vi "首页.vi"() -> ()   [LabVIEW 2016]
uses:
  <vilib>/Utility/miscctls.llb/LVPointTypeDef.ctl
  PLC/PLC.lvlib
  API/database/SQLite/SQLite Lib.lvlib
  API/database/Access/Access Lib.lvlib
panel:
  out "显示":T1
  out "动力环境":T3
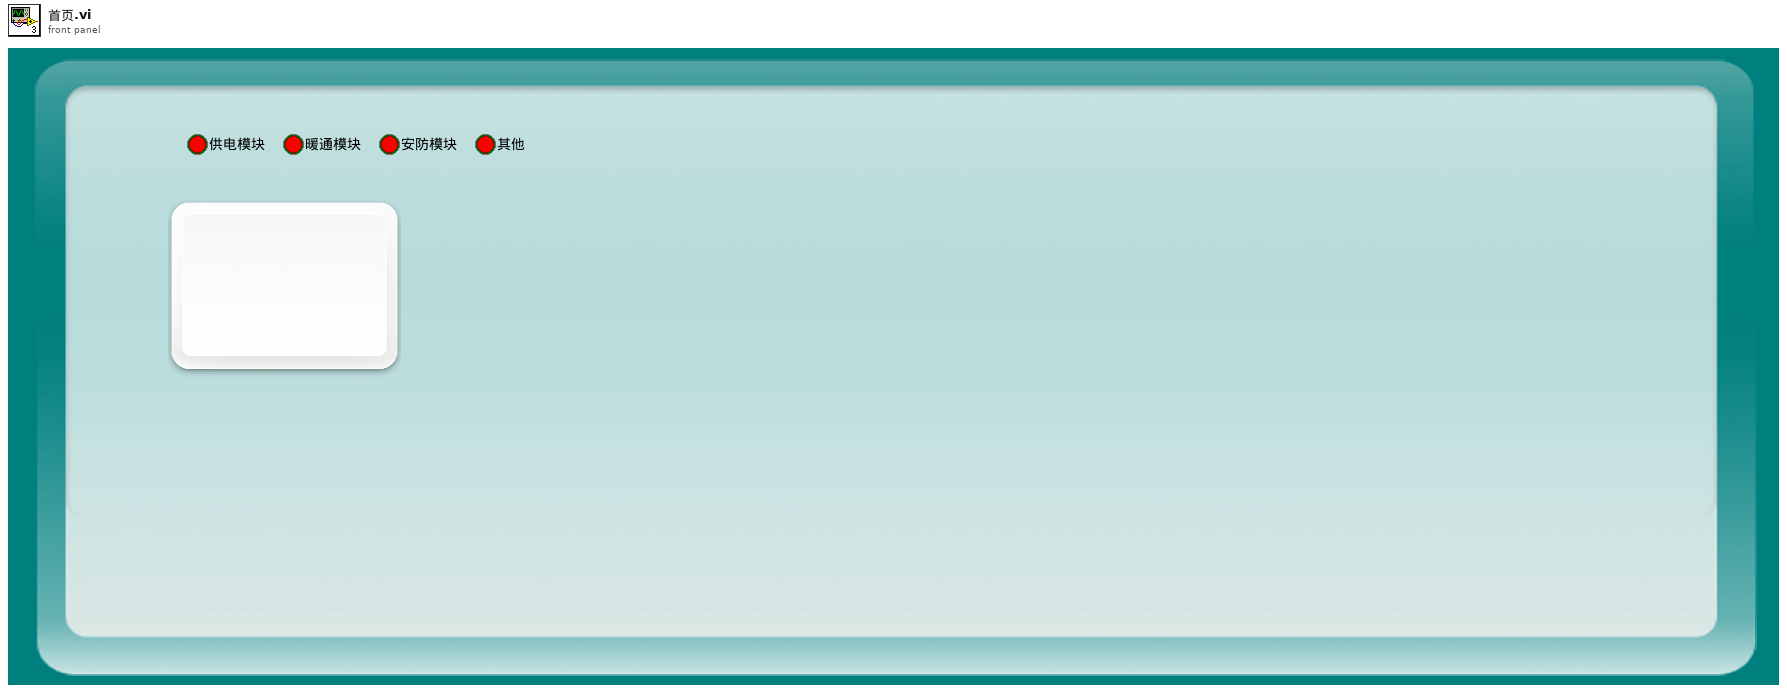
[diagram p1: front panel]
types:
  T1 = typedef "多数值显示.ctl" = cluster{"显示":T2, "显示 2":T2, "显示 3":T2, "显示 4":T2, "显示 5":T2, "显示 6":T2, "显示 12":T2, "显示 11":T2, "显示 10":T2, "显示 9":T2, "显示 8":T2, "显示 7":T2}
  T2 = typedef "数值显示.ctl" = cluster{"中文项目名称":string, "英文项目名称":string, "浓度":string, "单位":string}
  T3 = cluster{"供电模块":bool, "暖通模块":bool, "安防模块":bool, "其他":bool}
  T4 = typedef "LVPointTypeDef.ctl" = cluster{"Horizontal":i16, "Vertical":i16}
  T5 = cluster{"显示参数中文名":string, "显示参数英文名":string, "显示浓度":string, "显示单位":string}[]
  T6 = cluster{"显示参数中文名":string, "显示参数英文名":string, "显示浓度":string, "显示单位":string}
  T7 = typedef "数据库类型.ctl" = enum16{"Access", "SQLite"}
  T8 = cluster{"水温":bool, "pH":bool, "DO":bool, "Cond":bool, "Turb":bool, "氨氮":bool, "总磷":bool, "总氮":bool, "CODMn":bool, "CODCr":bool, "水位":bool, "流速":bool, "瞬时流量":bool, "ORP":bool, "氟化物":bool, "铅":bool, "镉":bool, "铜":bool, "锌":bool, "汞":bool, "叶绿素a":bool, "藻密度":bool, "氯化物":bool, "挥发酚":bool, "盐度":bool, "磷酸盐":bool, "硝氮":bool, "亚硝氮":bool, "硅酸盐":bool, "硫化物":bool, "余氯":bool}
  T9 = cluster{"AD0":sgl, "AD1":sgl, "AD2":sgl, "AD3":sgl, "AD4":sgl, "AD5":sgl}
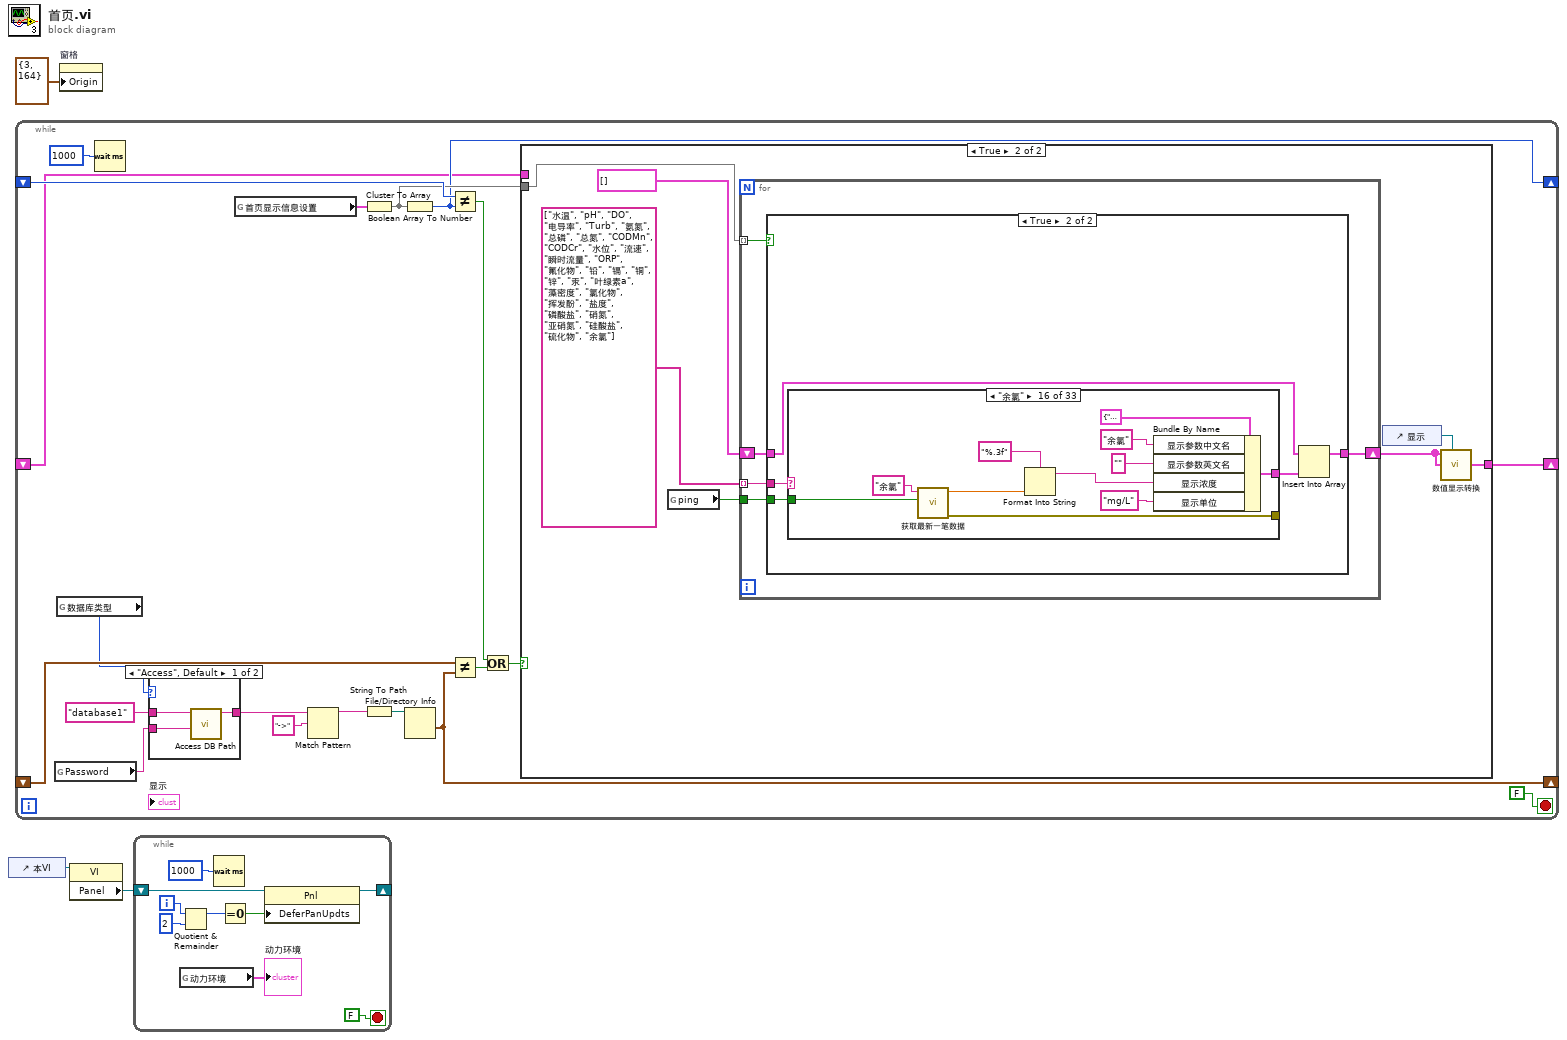
[diagram p0: block diagram]
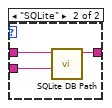
[diagram p2: hidden frame]
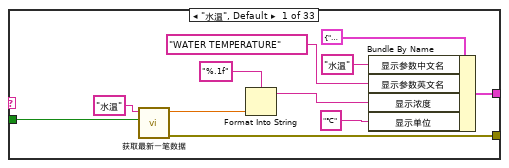
[diagram p5: hidden frame]
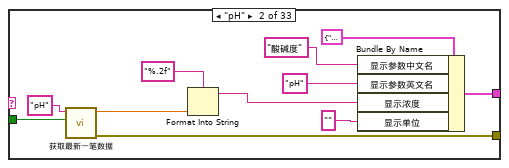
[diagram p6: hidden frame]
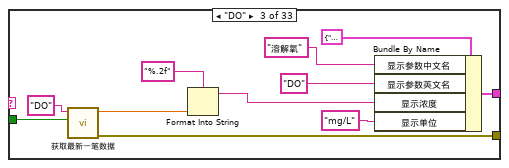
[diagram p7: hidden frame]
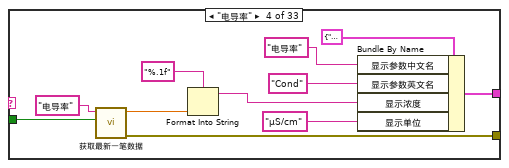
[diagram p8: hidden frame]
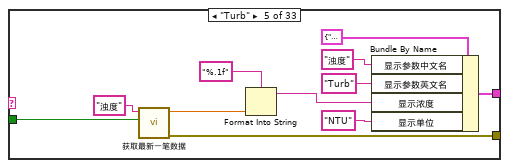
[diagram p9: hidden frame]
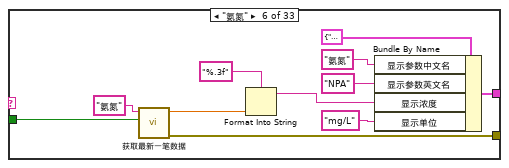
[diagram p10: hidden frame]
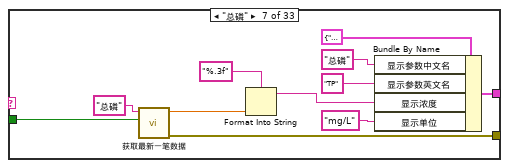
[diagram p11: hidden frame]
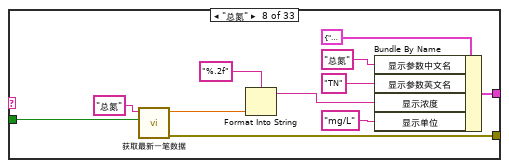
[diagram p12: hidden frame]
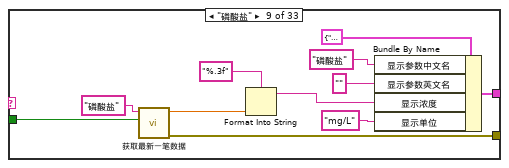
[diagram p13: hidden frame]
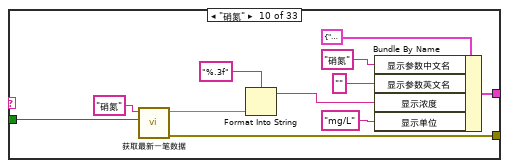
[diagram p14: hidden frame]
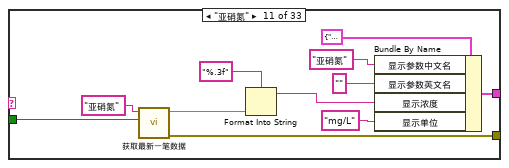
[diagram p15: hidden frame]
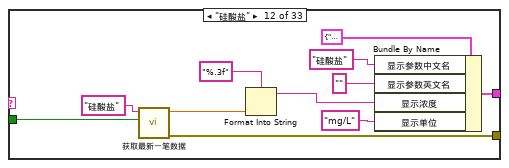
[diagram p16: hidden frame]
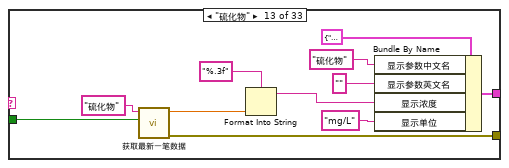
[diagram p17: hidden frame]
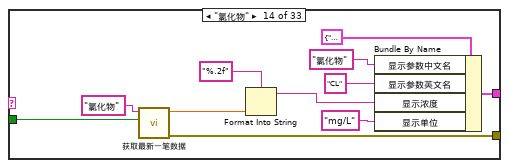
[diagram p18: hidden frame]
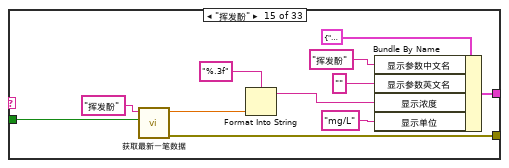
[diagram p19: hidden frame]
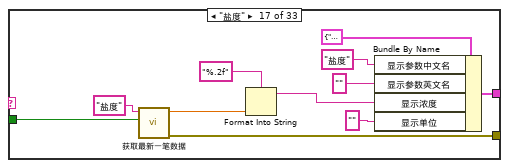
[diagram p20: hidden frame]
diagram:
  n1 = control-ref of="本VI"() -> (w2:refnum<vi>)
  n2 = while {
    shift-right: [w18] -> _
    shift-left: _ -> [w20]
    shift-right: [w6] -> _
    shift-left: _ -> [w17]
    shift-right: [w7] -> _
    shift-left: _ -> [w13]
    stop <- FALSE stop-if-true
    n3 = global read "非断电保持全局变量.vi" "Password"() -> (w4:string)
    n4 = global read "非断电保持全局变量.vi" "数据库类型"() -> (w5:T7)
    n5 = Wait (ms)(milliseconds to wait=u32 1000 ("等待时间（毫秒）")) -> ()  [unwired: 1 out]
    n6 = case shown="\"Access\", Default" w5 {
      tunnel: "database1" ("database") -> [w26 w29]
      tunnel: [w25 w28] -> w11
      tunnel: w4 -> [w24 w27]
      frame "Access", Default {
        n7 = call "Access DB Path.vi"("Password"=w24, "database"=w26) -> ("Path out"=w25:string)  [unwired: 8 in, 1 out]
      }
      frame "SQLite" {
        n8 = call "SQLite DB Path.vi"("Password"=w27, "database"=w29) -> ("Path out"=w28:string)  [unwired: 9 in]
      }
    }
    n9 = global read "系统设置全局变量.vi" "首页显示信息设置"() -> (w21:T8)
    n10 = Match Pattern(string=w11, regular expression="->" ("正则表达式")) -> (before substring=w9:string)  [unwired: 1 in, 3 out]
    n11 = Cluster To Array(cluster=w21) -> (array=w19:bool[])
    n12 = String To Path(string=w9) -> (path=w8:path)
    n13 = Boolean Array To Number(Boolean array=w19) -> (number=w18:u32)
    n14 = File/Directory Info(path=w8) -> (last mod=w6:timestamp)  [unwired: 1 in, 6 out]
    n15 = Not Equal?(x=w20, y=w18) -> (x != y?=w14:bool)
    n16 = Not Equal?(x=w17, y=w6) -> (x != y?=w16:bool)
    n17 = Or(x=w14, y=w16) -> (x .or. y?=w15:bool)
    n18 = case shown="True" w15 {
      tunnel: w19 -> [_ w34]
      tunnel: [w30 w31] -> w7
      tunnel: w13 -> [w30 _]
      frame False {
      }
      frame True {
        n19 = global read "全局变量.vi" "ping"() -> (w33:bool)
        n20 = for {
          tunnel: w34 -> [w41] mode=indexing
          tunnel: string[] ["水温", "pH", "DO", "电导率", "Turb", "氨氮", "总磷", "总氮", "CODMn", "CODCr", "水位", "流速", "瞬时流量", "ORP", "氟化物", "铅", "镉", "铜", "锌", "汞", "叶绿素a", "藻密度", "氯化物", "挥发酚", "盐度", "磷酸盐", "硝氮", "亚硝氮", "硅酸盐", "硫化物", "余氯"] -> [w40] mode=indexing
          shift-right: [w38] -> w31
          shift-left: T5 [] -> [w39]
          tunnel: w33 -> [w37]
          n21 = case shown="True" w41 {
            tunnel: w40 -> [_ w47]
            tunnel: w39 -> [w42 w46]
            tunnel: [w42 w45] -> w38
            tunnel: w37 -> [_ w43]
            frame False {
            }
            frame True {
              n22 = case shown="\"余氯\"" w47 {
                selector: w47 -> [_ _ _ _ _ _ _ _ _ _ _ _ _ _ _ _ _ _ _ _ _ _ _ _ w312 w322 w332 w342 _ _ _ _ _]
                tunnel: [w51 w65 w76 w87 w98 w109 w120 w131 w142 w153 w164 w175 w186 w197 w208 w219 w230 w241 w252 w263 w274 w285 w296 w307 w318 w328 w338 w348 w355 w363 w368 w380 w389] -> w44
                tunnel: [w52 w62 w73 w84 w95 w106 w117 w128 w139 w150 w161 w172 w183 w194 w205 w216 w227 w238 w249 w260 w271 w282 w293 w304 w315 w325 w335 w345 _ _ _ _ _] -> _
                tunnel: w43 -> [w48 w59 w70 w81 w92 w103 w114 w125 w136 w147 w158 w169 w180 w191 w202 w213 w224 w235 w246 w257 w268 w279 w290 w301 w313 w323 w333 w343 _ _ _ _ _]
                frame "水温", Default {
                  n23 = call "获取最新一笔数据.vi"("ping"=w48, "table"="水温") -> ("错误输出"=w52:errorcluster, "data"=w49:dbl)  [unwired: 7 in, 1 out]
                  n24 = Format Into String(format string="%.1f" ("格式字符串"), w49) -> (resulting string=w53:string)  [unwired: 2 in, 1 out]
                  n25 = Bundle By Name(cluster=T6 {"显示参数中文名"="", "显示参数英文名"="", "显示浓度"="", "显示单位"=""} ("元素"), "显示参数中文名"="水温", "显示参数英文名"="WATER TEMPERATURE", "显示浓度"=w53, "显示单位"="℃") -> (w51:T6)
                }
                frame "pH" {
                  n26 = call "获取最新一笔数据.vi"("ping"=w59, "table"="pH") -> ("错误输出"=w62:errorcluster, "data"=w60:dbl)  [unwired: 7 in, 1 out]
                  n27 = Format Into String(format string="%.2f" ("格式字符串"), w60) -> (resulting string=w63:string)  [unwired: 2 in, 1 out]
                  n28 = Bundle By Name(cluster=T6 {"显示参数中文名"="", "显示参数英文名"="", "显示浓度"="", "显示单位"=""} ("元素"), "显示参数中文名"="酸碱度", "显示参数英文名"="pH", "显示浓度"=w63, "显示单位"="") -> (w65:T6)
                }
                frame "DO" {
                  n29 = call "获取最新一笔数据.vi"("ping"=w70, "table"="DO") -> ("错误输出"=w73:errorcluster, "data"=w71:dbl)  [unwired: 7 in, 1 out]
                  n30 = Format Into String(format string="%.2f" ("格式字符串"), w71) -> (resulting string=w74:string)  [unwired: 2 in, 1 out]
                  n31 = Bundle By Name(cluster=T6 {"显示参数中文名"="", "显示参数英文名"="", "显示浓度"="", "显示单位"=""} ("元素"), "显示参数中文名"="溶解氧", "显示参数英文名"="DO", "显示浓度"=w74, "显示单位"="mg/L") -> (w76:T6)
                }
                frame "电导率" {
                  n32 = call "获取最新一笔数据.vi"("ping"=w81, "table"="电导率") -> ("错误输出"=w84:errorcluster, "data"=w82:dbl)  [unwired: 7 in, 1 out]
                  n33 = Format Into String(format string="%.1f" ("格式字符串"), w82) -> (resulting string=w85:string)  [unwired: 2 in, 1 out]
                  n34 = Bundle By Name(cluster=T6 {"显示参数中文名"="", "显示参数英文名"="", "显示浓度"="", "显示单位"=""} ("元素"), "显示参数中文名"="电导率", "显示参数英文名"="Cond", "显示浓度"=w85, "显示单位"="μS/cm") -> (w87:T6)
                }
                frame "Turb" {
                  n35 = call "获取最新一笔数据.vi"("ping"=w92, "table"="浊度") -> ("错误输出"=w95:errorcluster, "data"=w93:dbl)  [unwired: 7 in, 1 out]
                  n36 = Format Into String(format string="%.1f" ("格式字符串"), w93) -> (resulting string=w96:string)  [unwired: 2 in, 1 out]
                  n37 = Bundle By Name(cluster=T6 {"显示参数中文名"="", "显示参数英文名"="", "显示浓度"="", "显示单位"=""} ("元素"), "显示参数中文名"="浊度", "显示参数英文名"="Turb", "显示浓度"=w96, "显示单位"="NTU") -> (w98:T6)
                }
                frame "氨氮" {
                  n38 = call "获取最新一笔数据.vi"("ping"=w103, "table"="氨氮") -> ("错误输出"=w106:errorcluster, "data"=w105:dbl)  [unwired: 7 in, 1 out]
                  n39 = Format Into String(format string="%.3f" ("格式字符串"), w105) -> (resulting string=w107:string)  [unwired: 2 in, 1 out]
                  n40 = Bundle By Name(cluster=T6 {"显示参数中文名"="", "显示参数英文名"="", "显示浓度"="", "显示单位"=""} ("元素"), "显示参数中文名"="氨氮", "显示参数英文名"="NPA", "显示浓度"=w107, "显示单位"="mg/L") -> (w109:T6)
                }
                frame "总磷" {
                  n41 = call "获取最新一笔数据.vi"("ping"=w114, "table"="总磷") -> ("错误输出"=w117:errorcluster, "data"=w116:dbl)  [unwired: 7 in, 1 out]
                  n42 = Format Into String(format string="%.3f" ("格式字符串"), w116) -> (resulting string=w118:string)  [unwired: 2 in, 1 out]
                  n43 = Bundle By Name(cluster=T6 {"显示参数中文名"="", "显示参数英文名"="", "显示浓度"="", "显示单位"=""} ("元素"), "显示参数中文名"="总磷", "显示参数英文名"="TP", "显示浓度"=w118, "显示单位"="mg/L") -> (w120:T6)
                }
                frame "总氮" {
                  n44 = call "获取最新一笔数据.vi"("ping"=w125, "table"="总氮") -> ("错误输出"=w128:errorcluster, "data"=w127:dbl)  [unwired: 7 in, 1 out]
                  n45 = Format Into String(format string="%.2f" ("格式字符串"), w127) -> (resulting string=w129:string)  [unwired: 2 in, 1 out]
                  n46 = Bundle By Name(cluster=T6 {"显示参数中文名"="", "显示参数英文名"="", "显示浓度"="", "显示单位"=""} ("元素"), "显示参数中文名"="总氮", "显示参数英文名"="TN", "显示浓度"=w129, "显示单位"="mg/L") -> (w131:T6)
                }
                frame "磷酸盐" {
                  n47 = call "获取最新一笔数据.vi"("ping"=w136, "table"="磷酸盐") -> ("错误输出"=w139:errorcluster, "data"=w138:dbl)  [unwired: 7 in, 1 out]
                  n48 = Format Into String(format string="%.3f" ("格式字符串"), w138) -> (resulting string=w140:string)  [unwired: 2 in, 1 out]
                  n49 = Bundle By Name(cluster=T6 {"显示参数中文名"="", "显示参数英文名"="", "显示浓度"="", "显示单位"=""} ("元素"), "显示参数中文名"="磷酸盐", "显示参数英文名"="", "显示浓度"=w140, "显示单位"="mg/L") -> (w142:T6)
                }
                frame "硝氮" {
                  n50 = call "获取最新一笔数据.vi"("ping"=w147, "table"="硝氮") -> ("错误输出"=w150:errorcluster, "data"=w149:dbl)  [unwired: 7 in, 1 out]
                  n51 = Format Into String(format string="%.3f" ("格式字符串"), w149) -> (resulting string=w151:string)  [unwired: 2 in, 1 out]
                  n52 = Bundle By Name(cluster=T6 {"显示参数中文名"="", "显示参数英文名"="", "显示浓度"="", "显示单位"=""} ("元素"), "显示参数中文名"="硝氮", "显示参数英文名"="", "显示浓度"=w151, "显示单位"="mg/L") -> (w153:T6)
                }
                frame "亚硝氮" {
                  n53 = call "获取最新一笔数据.vi"("ping"=w158, "table"="亚硝氮") -> ("错误输出"=w161:errorcluster, "data"=w160:dbl)  [unwired: 7 in, 1 out]
                  n54 = Format Into String(format string="%.3f" ("格式字符串"), w160) -> (resulting string=w162:string)  [unwired: 2 in, 1 out]
                  n55 = Bundle By Name(cluster=T6 {"显示参数中文名"="", "显示参数英文名"="", "显示浓度"="", "显示单位"=""} ("元素"), "显示参数中文名"="亚硝氮", "显示参数英文名"="", "显示浓度"=w162, "显示单位"="mg/L") -> (w164:T6)
                }
                frame "硅酸盐" {
                  n56 = call "获取最新一笔数据.vi"("ping"=w169, "table"="硅酸盐") -> ("错误输出"=w172:errorcluster, "data"=w171:dbl)  [unwired: 7 in, 1 out]
                  n57 = Format Into String(format string="%.3f" ("格式字符串"), w171) -> (resulting string=w173:string)  [unwired: 2 in, 1 out]
                  n58 = Bundle By Name(cluster=T6 {"显示参数中文名"="", "显示参数英文名"="", "显示浓度"="", "显示单位"=""} ("元素"), "显示参数中文名"="硅酸盐", "显示参数英文名"="", "显示浓度"=w173, "显示单位"="mg/L") -> (w175:T6)
                }
                frame "硫化物" {
                  n59 = call "获取最新一笔数据.vi"("ping"=w180, "table"="硫化物") -> ("错误输出"=w183:errorcluster, "data"=w182:dbl)  [unwired: 7 in, 1 out]
                  n60 = Format Into String(format string="%.3f" ("格式字符串"), w182) -> (resulting string=w184:string)  [unwired: 2 in, 1 out]
                  n61 = Bundle By Name(cluster=T6 {"显示参数中文名"="", "显示参数英文名"="", "显示浓度"="", "显示单位"=""} ("元素"), "显示参数中文名"="硫化物", "显示参数英文名"="", "显示浓度"=w184, "显示单位"="mg/L") -> (w186:T6)
                }
                frame "氯化物" {
                  n62 = call "获取最新一笔数据.vi"("ping"=w191, "table"="氯化物") -> ("错误输出"=w194:errorcluster, "data"=w193:dbl)  [unwired: 7 in, 1 out]
                  n63 = Format Into String(format string="%.2f" ("格式字符串"), w193) -> (resulting string=w195:string)  [unwired: 2 in, 1 out]
                  n64 = Bundle By Name(cluster=T6 {"显示参数中文名"="", "显示参数英文名"="", "显示浓度"="", "显示单位"=""} ("元素"), "显示参数中文名"="氯化物", "显示参数英文名"="CL", "显示浓度"=w195, "显示单位"="mg/L") -> (w197:T6)
                }
                frame "挥发酚" {
                  n65 = call "获取最新一笔数据.vi"("ping"=w202, "table"="挥发酚") -> ("错误输出"=w205:errorcluster, "data"=w204:dbl)  [unwired: 7 in, 1 out]
                  n66 = Format Into String(format string="%.3f" ("格式字符串"), w204) -> (resulting string=w206:string)  [unwired: 2 in, 1 out]
                  n67 = Bundle By Name(cluster=T6 {"显示参数中文名"="", "显示参数英文名"="", "显示浓度"="", "显示单位"=""} ("元素"), "显示参数中文名"="挥发酚", "显示参数英文名"="", "显示浓度"=w206, "显示单位"="mg/L") -> (w208:T6)
                }
                frame "余氯" {
                  n68 = call "获取最新一笔数据.vi"("ping"=w213, "table"="余氯") -> ("错误输出"=w216:errorcluster, "data"=w215:dbl)  [unwired: 7 in, 1 out]
                  n69 = Format Into String(format string="%.3f" ("格式字符串"), w215) -> (resulting string=w217:string)  [unwired: 2 in, 1 out]
                  n70 = Bundle By Name(cluster=T6 {"显示参数中文名"="", "显示参数英文名"="", "显示浓度"="", "显示单位"=""} ("元素"), "显示参数中文名"="余氯", "显示参数英文名"="", "显示浓度"=w217, "显示单位"="mg/L") -> (w219:T6)
                }
                frame "盐度" {
                  n71 = call "获取最新一笔数据.vi"("ping"=w224, "table"="盐度") -> ("错误输出"=w227:errorcluster, "data"=w226:dbl)  [unwired: 7 in, 1 out]
                  n72 = Format Into String(format string="%.2f" ("格式字符串"), w226) -> (resulting string=w228:string)  [unwired: 2 in, 1 out]
                  n73 = Bundle By Name(cluster=T6 {"显示参数中文名"="", "显示参数英文名"="", "显示浓度"="", "显示单位"=""} ("元素"), "显示参数中文名"="盐度", "显示参数英文名"="", "显示浓度"=w228, "显示单位"="") -> (w230:T6)
                }
                frame "CODMn" {
                  n74 = call "获取最新一笔数据.vi"("ping"=w235, "table"="CODmn") -> ("错误输出"=w238:errorcluster, "data"=w237:dbl)  [unwired: 7 in, 1 out]
                  n75 = Format Into String(format string="%.2f" ("格式字符串"), w237) -> (resulting string=w239:string)  [unwired: 2 in, 1 out]
                  n76 = Bundle By Name(cluster=T6 {"显示参数中文名"="", "显示参数英文名"="", "显示浓度"="", "显示单位"=""} ("元素"), "显示参数中文名"="高锰酸盐指数", "显示参数英文名"="CODmn", "显示浓度"=w239, "显示单位"="mg/L") -> (w241:T6)
                }
                frame "CODCr" {
                  n77 = call "获取最新一笔数据.vi"("ping"=w246, "table"="CODCr") -> ("错误输出"=w249:errorcluster, "data"=w248:dbl)  [unwired: 7 in, 1 out]
                  n78 = Format Into String(format string="%.2f" ("格式字符串"), w248) -> (resulting string=w250:string)  [unwired: 2 in, 1 out]
                  n79 = Bundle By Name(cluster=T6 {"显示参数中文名"="", "显示参数英文名"="", "显示浓度"="", "显示单位"=""} ("元素"), "显示参数中文名"="化学需氧量", "显示参数英文名"="CODCr", "显示浓度"=w250, "显示单位"="mg/L") -> (w252:T6)
                }
                frame "氟化物" {
                  n80 = call "获取最新一笔数据.vi"("ping"=w257, "table"="氟化物") -> ("错误输出"=w260:errorcluster, "data"=w259:dbl)  [unwired: 7 in, 1 out]
                  n81 = Format Into String(format string="%.2f" ("格式字符串"), w259) -> (resulting string=w261:string)  [unwired: 2 in, 1 out]
                  n82 = Bundle By Name(cluster=T6 {"显示参数中文名"="", "显示参数英文名"="", "显示浓度"="", "显示单位"=""} ("元素"), "显示参数中文名"="氟化物", "显示参数英文名"="F", "显示浓度"=w261, "显示单位"="mg/L") -> (w263:T6)
                }
                frame "叶绿素a" {
                  n83 = call "获取最新一笔数据.vi"("ping"=w268, "table"="叶绿素a") -> ("错误输出"=w271:errorcluster, "data"=w270:dbl)  [unwired: 7 in, 1 out]
                  n84 = Format Into String(format string="%.2f" ("格式字符串"), w270) -> (resulting string=w272:string)  [unwired: 2 in, 1 out]
                  n85 = Bundle By Name(cluster=T6 {"显示参数中文名"="", "显示参数英文名"="", "显示浓度"="", "显示单位"=""} ("元素"), "显示参数中文名"="叶绿素a", "显示参数英文名"="Chla", "显示浓度"=w272, "显示单位"="μg/L") -> (w274:T6)
                }
                frame "藻密度" {
                  n86 = call "获取最新一笔数据.vi"("ping"=w279, "table"="藻密度") -> ("错误输出"=w282:errorcluster, "data"=w281:dbl)  [unwired: 7 in, 1 out]
                  n87 = Format Into String(format string="%.1f" ("格式字符串"), w281) -> (resulting string=w283:string)  [unwired: 2 in, 1 out]
                  n88 = Bundle By Name(cluster=T6 {"显示参数中文名"="", "显示参数英文名"="", "显示浓度"="", "显示单位"=""} ("元素"), "显示参数中文名"="藻密度", "显示参数英文名"="Algae", "显示浓度"=w283, "显示单位"="cells/mL") -> (w285:T6)
                }
                frame "ORP" {
                  n89 = call "获取最新一笔数据.vi"("ping"=w290, "table"="ORP") -> ("错误输出"=w293:errorcluster, "data"=w292:dbl)  [unwired: 7 in, 1 out]
                  n90 = Format Into String(format string="%.2f" ("格式字符串"), w292) -> (resulting string=w294:string)  [unwired: 2 in, 1 out]
                  n91 = Bundle By Name(cluster=T6 {"显示参数中文名"="", "显示参数英文名"="", "显示浓度"="", "显示单位"=""} ("元素"), "显示参数中文名"="氧化还原电位", "显示参数英文名"="ORP", "显示浓度"=w294, "显示单位"="mV") -> (w296:T6)
                }
                frame "铅" {
                  n92 = call "获取最新一笔数据.vi"("ping"=w301, "table"="铅") -> ("错误输出"=w304:errorcluster, "data"=w303:dbl)  [unwired: 7 in, 1 out]
                  n93 = Format Into String(format string="%.6f" ("格式字符串"), w303) -> (resulting string=w305:string)  [unwired: 2 in, 1 out]
                  n94 = Bundle By Name(cluster=T6 {"显示参数中文名"="", "显示参数英文名"="", "显示浓度"="", "显示单位"=""} ("元素"), "显示参数中文名"="铅", "显示参数英文名"="Pb", "显示浓度"=w305, "显示单位"="mg/L") -> (w307:T6)
                }
                frame "镉" {
                  n95 = call "获取最新一笔数据.vi"("ping"=w313, "table"=w312) -> ("错误输出"=w315:errorcluster, "data"=w314:dbl)  [unwired: 7 in, 1 out]
                  n96 = Format Into String(format string="%.6f" ("格式字符串"), w314) -> (resulting string=w316:string)  [unwired: 2 in, 1 out]
                  n97 = Bundle By Name(cluster=T6 {"显示参数中文名"="", "显示参数英文名"="", "显示浓度"="", "显示单位"=""} ("元素"), "显示参数中文名"=w312, "显示参数英文名"="Cd", "显示浓度"=w316, "显示单位"="mg/L") -> (w318:T6)
                }
                frame "铜" {
                  n98 = call "获取最新一笔数据.vi"("ping"=w323, "table"=w322) -> ("错误输出"=w325:errorcluster, "data"=w324:dbl)  [unwired: 7 in, 1 out]
                  n99 = Format Into String(format string="%.6f" ("格式字符串"), w324) -> (resulting string=w326:string)  [unwired: 2 in, 1 out]
                  n100 = Bundle By Name(cluster=T6 {"显示参数中文名"="", "显示参数英文名"="", "显示浓度"="", "显示单位"=""} ("元素"), "显示参数中文名"=w322, "显示参数英文名"="Cu", "显示浓度"=w326, "显示单位"="mg/L") -> (w328:T6)
                }
                frame "锌" {
                  n101 = call "获取最新一笔数据.vi"("ping"=w333, "table"=w332) -> ("错误输出"=w335:errorcluster, "data"=w334:dbl)  [unwired: 7 in, 1 out]
                  n102 = Format Into String(format string="%.6f" ("格式字符串"), w334) -> (resulting string=w336:string)  [unwired: 2 in, 1 out]
                  n103 = Bundle By Name(cluster=T6 {"显示参数中文名"="", "显示参数英文名"="", "显示浓度"="", "显示单位"=""} ("元素"), "显示参数中文名"=w332, "显示参数英文名"="Zn", "显示浓度"=w336, "显示单位"="mg/L") -> (w338:T6)
                }
                frame "总汞" {
                  n104 = call "获取最新一笔数据.vi"("ping"=w343, "table"=w342) -> ("错误输出"=w345:errorcluster, "data"=w344:dbl)  [unwired: 7 in, 1 out]
                  n105 = Format Into String(format string="%.6f" ("格式字符串"), w344) -> (resulting string=w346:string)  [unwired: 2 in, 1 out]
                  n106 = Bundle By Name(cluster=T6 {"显示参数中文名"="", "显示参数英文名"="", "显示浓度"="", "显示单位"=""} ("元素"), "显示参数中文名"=w342, "显示参数英文名"="Hg", "显示浓度"=w346, "显示单位"="mg/L") -> (w348:T6)
                }
                frame "水位" {
                  n107 = global read "流量计全局变量.vi" "平均水位"() -> (w352:dbl)
                  n108 = Format Into String(format string="%.2f" ("格式字符串"), w352) -> (resulting string=w353:string)  [unwired: 2 in, 1 out]
                  n109 = Bundle By Name(cluster=T6 {"显示参数中文名"="", "显示参数英文名"="", "显示浓度"="", "显示单位"=""} ("元素"), "显示参数中文名"="水位", "显示参数英文名"="WaterLevel", "显示浓度"=w353, "显示单位"="m") -> (w355:T6)
                }
                frame "流速" {
                  n110 = global read "流量计全局变量.vi" "平均流速"() -> (w360:dbl)
                  n111 = Format Into String(format string="%.2f" ("格式字符串"), w360) -> (resulting string=w361:string)  [unwired: 2 in, 1 out]
                  n112 = Bundle By Name(cluster=T6 {"显示参数中文名"="", "显示参数英文名"="", "显示浓度"="", "显示单位"=""} ("元素"), "显示参数中文名"="流速", "显示参数英文名"="FlowRate", "显示浓度"=w361, "显示单位"="m/s") -> (w363:T6)
                }
                frame "瞬时流量" {
                  n113 = global read "流量计全局变量.vi" "总流量"() -> (w369:dbl)
                  n114 = Format Into String(format string="%.2f" ("格式字符串"), w369) -> (resulting string=w370:string)  [unwired: 2 in, 1 out]
                  n115 = Bundle By Name(cluster=T6 {"显示参数中文名"="", "显示参数英文名"="", "显示浓度"="", "显示单位"=""} ("元素"), "显示参数中文名"="瞬时流量", "显示参数英文名"="InstantaneousFlow", "显示浓度"=w370, "显示单位"="m3/s") -> (w368:T6)
                }
                frame "湿度" {
                  n116 = global read "采配水全局变量.vi" "转换值"() -> (w377:T9)
                  n117 = Unbundle By Name(w377) -> ("AD1"=w379:sgl)
                  n118 = Format Into String(format string="%.2f" ("格式字符串"), w379) -> (resulting string=w376:string)  [unwired: 2 in, 1 out]
                  n119 = Bundle By Name(cluster=T6 {"显示参数中文名"="", "显示参数英文名"="", "显示浓度"="", "显示单位"=""} ("元素"), "显示参数中文名"="湿度", "显示参数英文名"="HUMIDITY", "显示浓度"=w376, "显示单位"="%") -> (w380:T6)
                }
                frame "室温" {
                  n120 = global read "采配水全局变量.vi" "转换值"() -> (w386:T9)
                  n121 = Unbundle By Name(w386) -> ("AD0"=w388:sgl)
                  n122 = Format Into String(format string="%.2f" ("格式字符串"), w388) -> (resulting string=w385:string)  [unwired: 2 in, 1 out]
                  n123 = Bundle By Name(cluster=T6 {"显示参数中文名"="", "显示参数英文名"="", "显示浓度"="", "显示单位"=""} ("元素"), "显示参数中文名"="室温", "显示参数英文名"="TEMPERATURE", "显示浓度"=w385, "显示单位"="℃") -> (w389:T6)
                }
              }
              n124 = Insert Into Array(array=w46, new element=w44) -> (w45:T5)  [unwired: 1 in]
            }
          }
        }
        n125 = control-ref of="显示"() -> (w32:refnum<vi>)
        n126 = call "数值显示转换.vi"("显示"=w32, "数组"=w31) -> ()  [unwired: 10 in]
      }
    }
  }
  n127 = property on="窗格" class="Pane"("Origin"=T4 {"Horizontal"=3, "Vertical"=164} ("原点")) -> ()  [unwired: 2 in, 2 out]
  n128 = property class="VI"(reference=w2) -> ("Panel"=w1:refnum<vi>)  [unwired: 1 in, 2 out]
  n129 = while {
    shift-right: [w394] -> _
    shift-left: w1 -> [w399]
    i -> [w398]
    stop <- FALSE stop-if-true
    n130 = global read "外部交互全局变量.vi" "动力环境"() -> (→"动力环境":T3)
    n131 = Quotient & Remainder(x=w398, y=2) -> (x-y*floor(x/y)=w396:i32)  [unwired: 1 out]
    n132 = Wait (ms)(milliseconds to wait=u32 1000 ("等待时间（毫秒）")) -> ()  [unwired: 1 out]
    n133 = Equal To 0?(x=w396) -> (x = 0?=w395:bool)
    n134 = property class="Pnl"(reference=w399, "DeferPanUpdts"=w395) -> (reference out=w394:refnum<vi>)  [unwired: 1 in, 1 out]
  }
